vi "main.vi"() -> ()   [LabVIEW 2015]
uses:
  Solution/Controls/Zone Setup.ctl
  Solution/Controls/Zone.ctl
  Solution/Controls/Zone Indicators.ctl
  controls/state.ctl
  controls/sprinkler data.ctl
  controls/timer state.ctl
panel:
  out "error out":errorcluster
  in  "error in":errorcluster
  out "Controller Status":string
  in  "Simulation Controls":T1 {"Water Pressure Sensor (%)" scale=0.0..100.0}
  out "Zone Indicators":T2 {"Timing" format="%#.0g"}
  in  "Zone Setup Array":T3[](array[typedef])
  in  "Controls":T5
  # "Rain"
  # "No Rain"
  # "Continuous"
  # "Single"
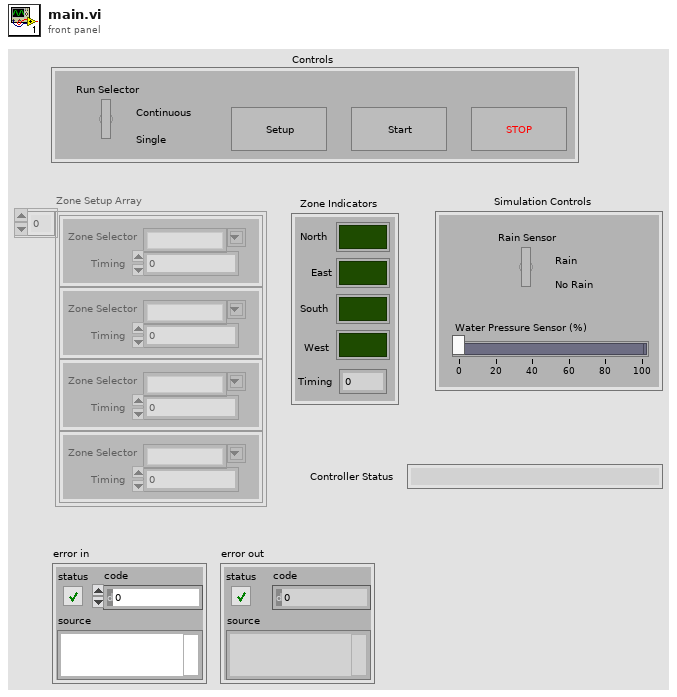
[diagram p1: front panel]
types:
  T1 = cluster{"Rain Sensor":bool, "Water Pressure Sensor (%)":dbl}
  T2 = typedef "Zone Indicators.ctl" = cluster{"North":bool, "East":bool, "South":bool, "West":bool, "Timing":dbl}
  T3 = typedef "Zone Setup.ctl" = cluster{"Zone Selector":T4, "Timing":u32}
  T4 = typedef "Zone.ctl" = string
  T5 = cluster{"Run Selector":bool, "Setup":bool, "Start":bool, "Stop":bool}
  T6 = typedef "state.ctl" = enum16{"Error", "End", "Start", "Exit", "Setup", "Low pressure", "Rain", "Run", "Idle", "Initialize"}
  T7 = enum8{"Enabled", "Disabled", "Disabled and Grayed Out"}
  T8 = typedef "timer state.ctl" = enum16{"Stop", "Start"}
  T9 = typedef "sprinkler data.ctl" = cluster{"Zone Setup Array":T3[], "Zone Indicators":T2, "order num":i32}
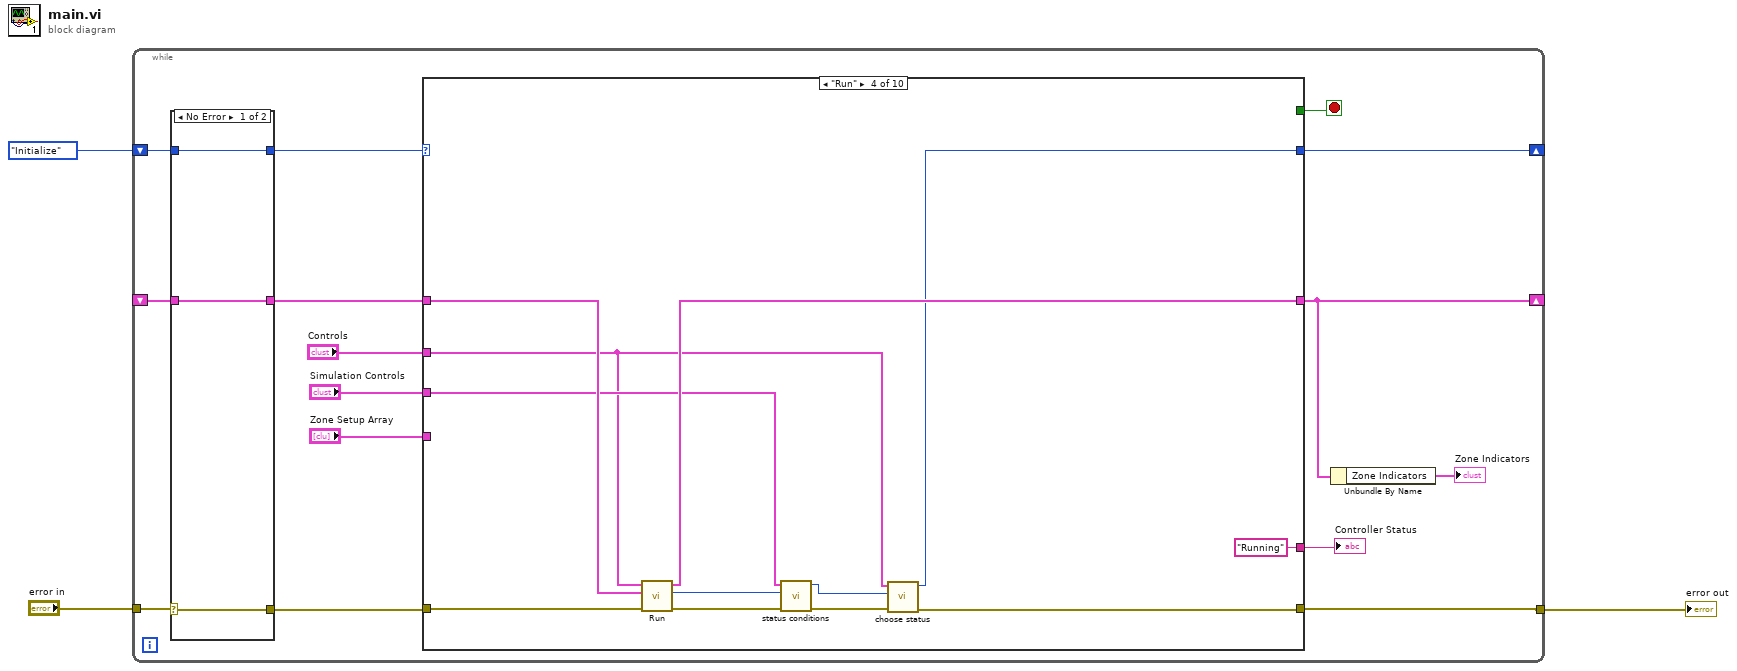
[diagram p0: block diagram]
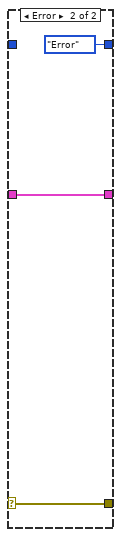
[diagram p2: hidden frame]
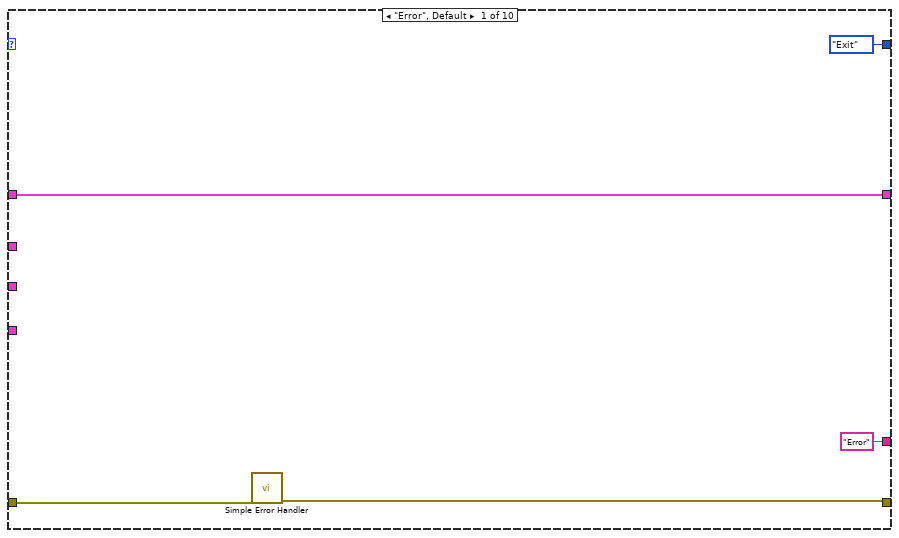
[diagram p3: hidden frame]
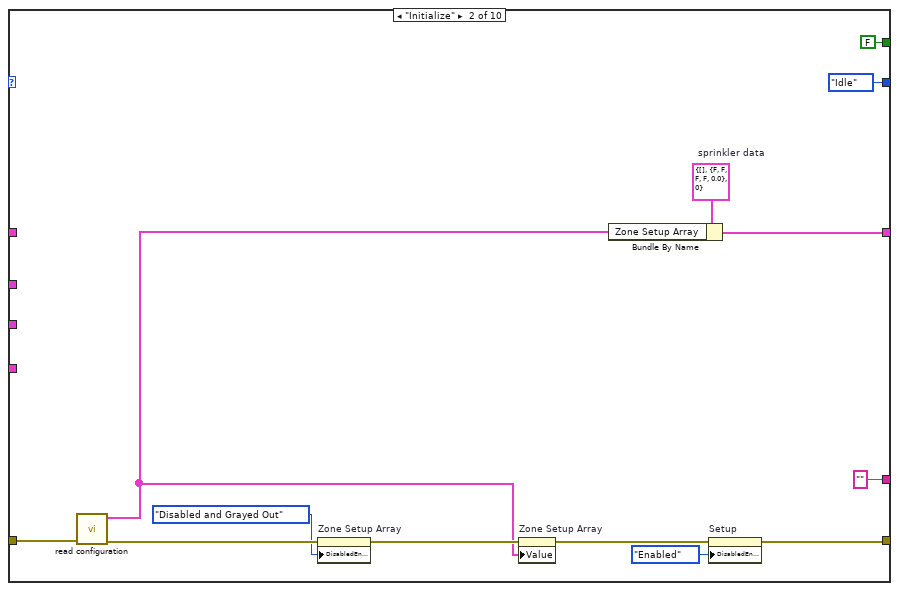
[diagram p4: hidden frame]
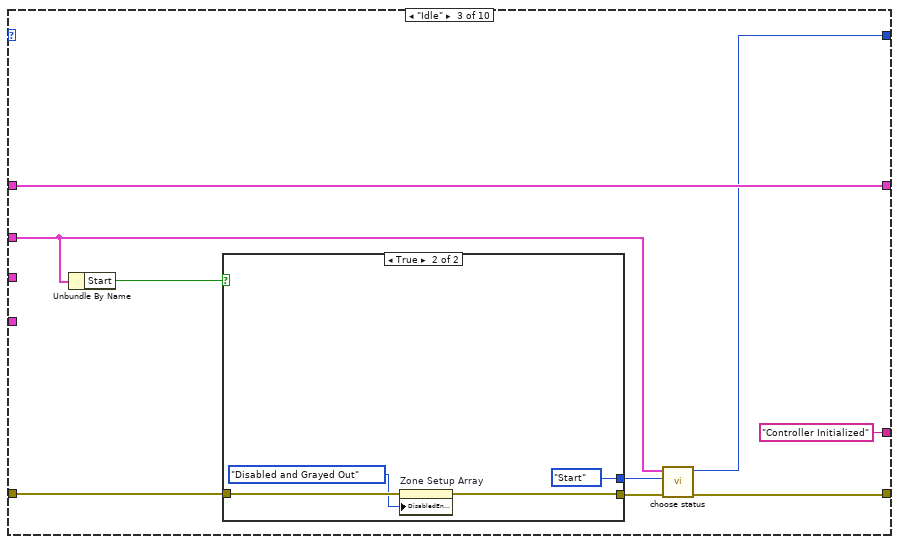
[diagram p5: hidden frame]
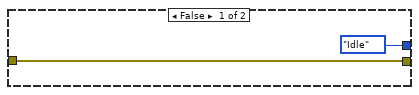
[diagram p6: hidden frame]
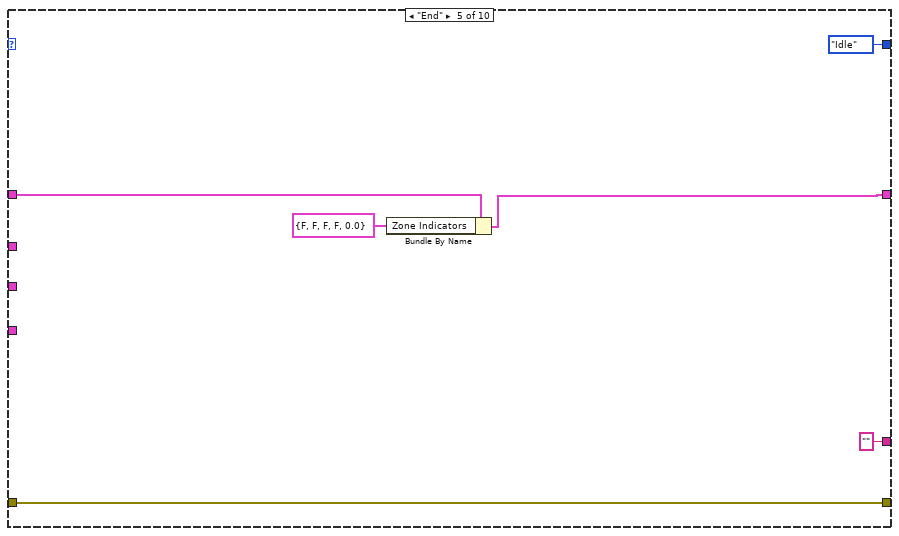
[diagram p7: hidden frame]
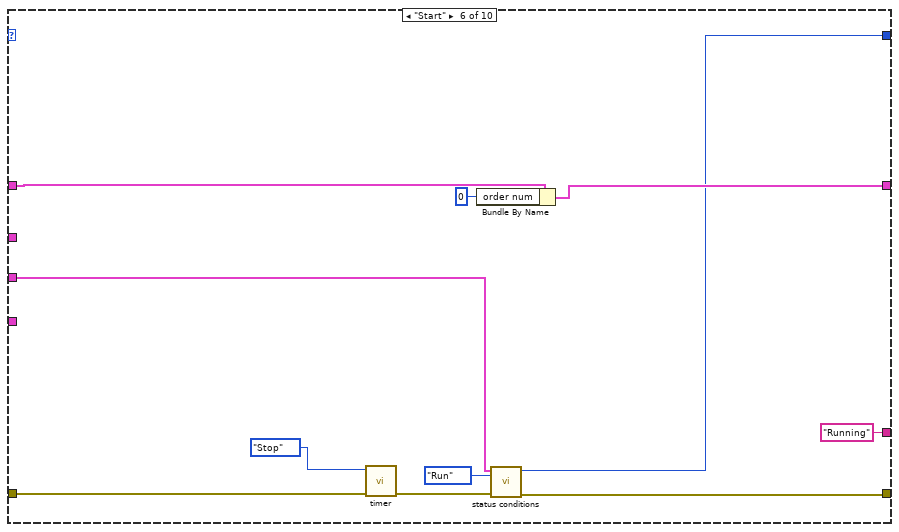
[diagram p8: hidden frame]
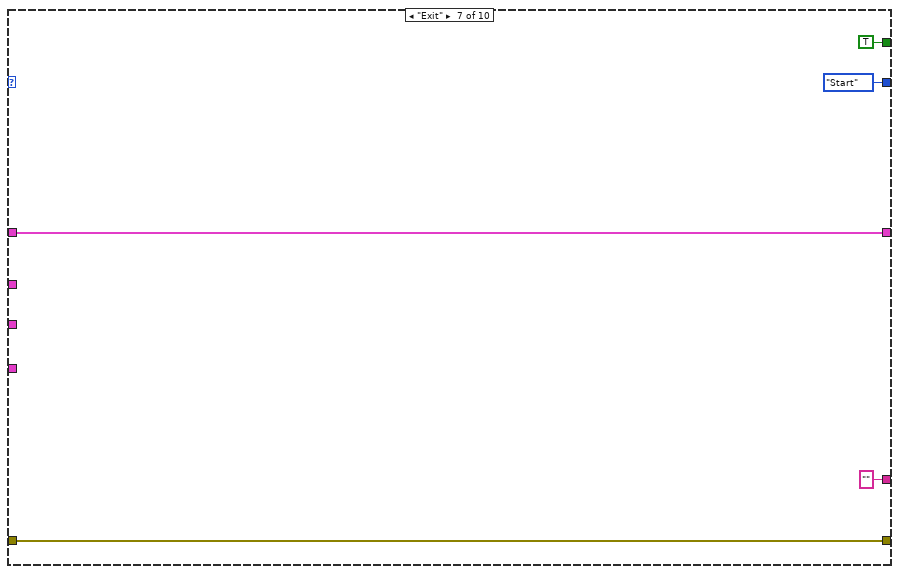
[diagram p9: hidden frame]
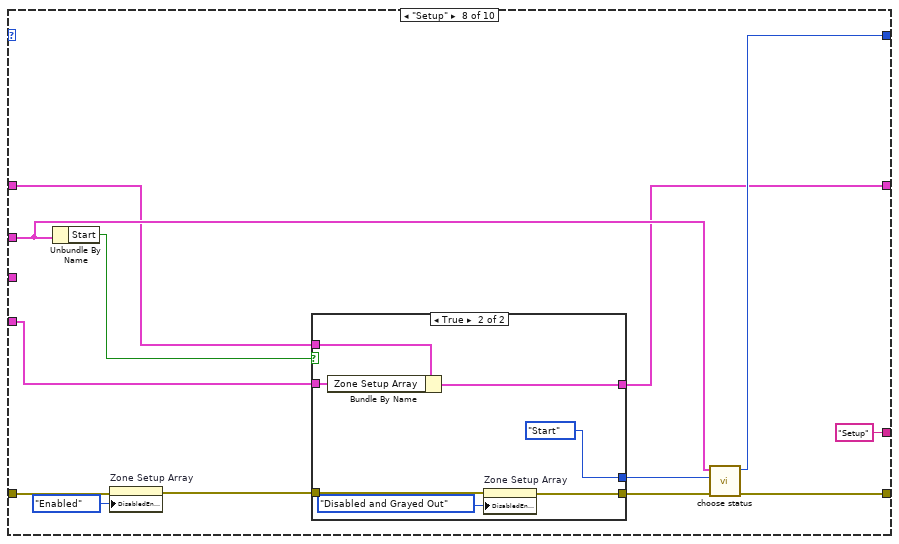
[diagram p10: hidden frame]
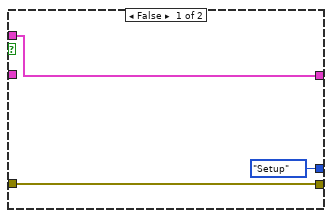
[diagram p11: hidden frame]
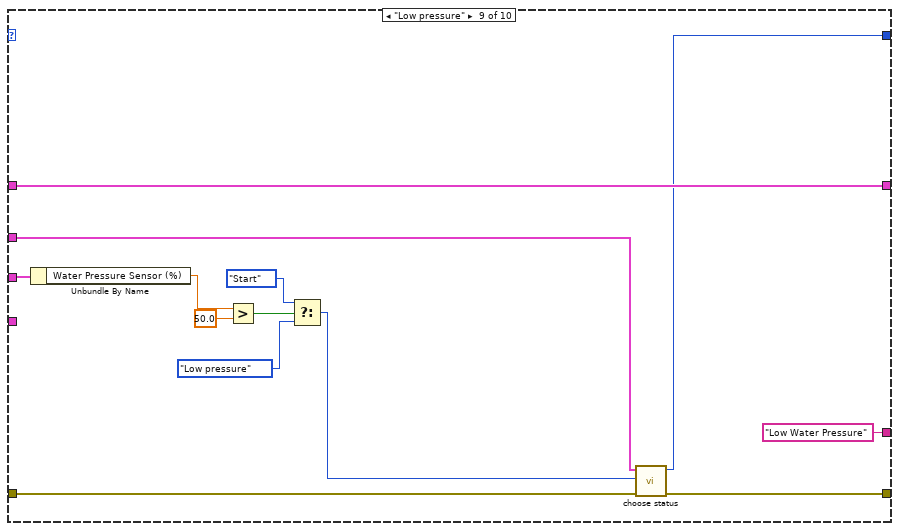
[diagram p12: hidden frame]
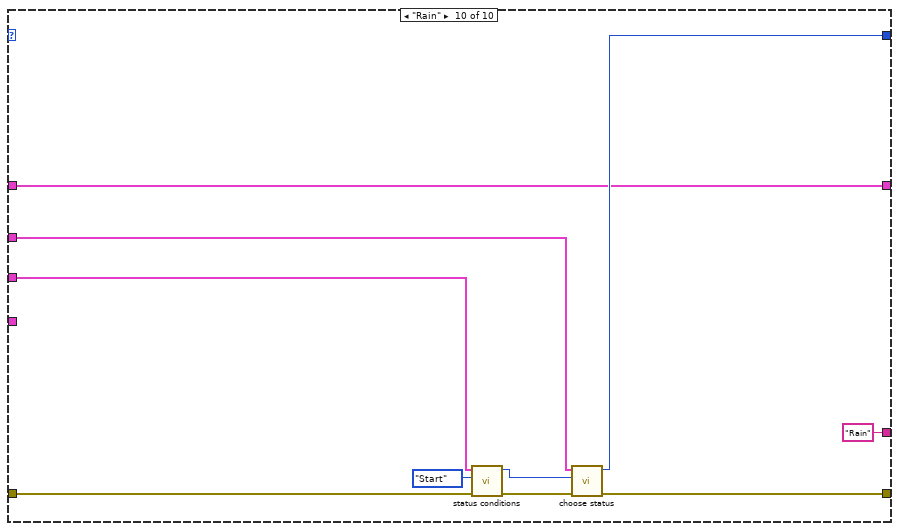
[diagram p13: hidden frame]
diagram:
  n1 = while {
    shift-right: [w13] -> _
    shift-left: state."Initialize" ("status") -> [w7]
    tunnel: "error in" -> [w10]
    tunnel: [w18] -> w1
    shift-right: [w12] -> _
    shift-left: _ -> [w8]
    stop <- w17 stop-if-true
    n2 = case shown="No Error" w10 {
      selector: w10 -> [w19 w23]
      tunnel: [w21 w24] -> w9
      tunnel: w8 -> [w21 w24]
      tunnel: w7 -> [w20 _]
      tunnel: [w20 state."Error" ("status out")] -> w6
      tunnel: [w19 w23] -> w5
      frame No Error {
      }
      frame Error {
      }
    }
    n3 = case shown="\"Run\"" w6 {
      tunnel: w5 -> [w29 w41 w50 w69 w70 w86 w88 w104 w127 w137]
      tunnel: [w28 w31 w47 w59 w70 w79 w88 w99 w126 w135] -> w18
      tunnel: [_ FALSE _ _ _ _ TRUE _ _ _] -> w17
      tunnel: [w26 w39 w49 w67 w73 w82 w89 w93 w123 w128] -> w12
      tunnel: ["Error" "" "Controller Initialized" "Running" "" "Running" "" "Setup" "Low Water Pressure" "Rain"] -> w16
      tunnel: w9 -> [w26 _ w49 w68 w75 w84 w89 w95 w123 w128]
      tunnel: "Controls" -> [_ _ w44 w62 _ _ _ w97 w124 w130]
      tunnel: "Simulation Controls" -> [_ _ _ w65 _ w78 _ _ w122 w133]
      tunnel: [state."Exit" ("status out") state."Idle" ("status out") w46 w60 state."Idle" ("status out") w76 state."Start" ("status out") w96 w115 w129] -> w13
      tunnel: "Zone Setup Array" -> [_ _ _ _ _ _ _ w94 _ _]
      frame "Error", Default {
        n4 = call <vilib>:"Simple Error Handler.vi"("error in (no error)"=w29) -> ("error out"=w28:errorcluster)  [unwired: 4 in, 4 out]
      }
      frame "Initialize" {
        w40 = T9 {"Zone Setup Array"=[], "Zone Indicators"={"North"=FALSE, "East"=FALSE, "South"=FALSE, "West"=FALSE, "Timing"=0.0}, "order num"=0}  # sprinkler data
        n5 = call "read configuration.vi"("error in (no error)"=w41) -> ("error out"=w38:errorcluster, "Zone Setup Array"=w33:T3[])  [unwired: 9 in]
        n6 = property on="Zone Setup Array" class="Arr (strict)"(error in=w38, "DisabledEnum"=T7."Disabled and Grayed Out" ("Disabled")) -> (error out=w34:errorcluster)  [unwired: 1 in, 1 out]
        n7 = property on="Zone Setup Array" class="Arr (strict)"(error in=w34, "Value"=w33) -> (error out=w32:errorcluster)  [unwired: 1 in, 1 out]
        n8 = Bundle By Name(cluster=w40, "Zone Setup Array"=w33) -> (w39:T9)
        n9 = property on="Setup" class="Bool"(error in=w32, "DisabledEnum"=T7."Enabled" ("Disabled")) -> (error out=w31:errorcluster)  [unwired: 1 in, 1 out]
      }
      frame "Idle" {
        n10 = Unbundle By Name(w44) -> ("Start"=w43:bool)
        n11 = case shown="True" w43 {
          tunnel: w50 -> [w52 w56]
          tunnel: [state."Idle" ("status") state."Start" ("status")] -> w45
          tunnel: [w52 w54] -> w48
          frame False {
          }
          frame True {
            n12 = property on="Zone Setup Array" class="Arr (strict)"(error in=w56, "DisabledEnum"=T7."Disabled and Grayed Out" ("Disabled")) -> (error out=w54:errorcluster)  [unwired: 1 in, 1 out]
          }
        }
        n13 = call "choose status.vi"("error in"=w48, "status in"=w45, "Controls"=w44) -> ("error out"=w47:errorcluster, "status out"=w46:T6)  [unwired: 7 in]
      }
      frame "Run" {
        n14 = call "Run.vi"("error in (no error)"=w69, "sprinkler data"=w68, "Controls"=w62) -> ("error out"=w66:errorcluster, "status"=w64:T6, "sprinkler data out"=w67:T9)  [unwired: 6 in]
        n15 = call "status conditions.vi"("error in"=w66, "status"=w64, "Simulation Controls"=w65) -> ("error out"=w61:errorcluster, "status out"=w63:T6)  [unwired: 7 in]
        n16 = call "choose status.vi"("error in"=w61, "status in"=w63, "Controls"=w62) -> ("error out"=w59:errorcluster, "status out"=w60:T6)  [unwired: 7 in]
      }
      frame "End" {
        n17 = Bundle By Name(cluster=w75, "Zone Indicators"=T2 {"North"=FALSE, "East"=FALSE, "South"=FALSE, "West"=FALSE, "Timing"=0.0}) -> (w73:T9)
      }
      frame "Start" {
        n18 = call "timer.vi"("error in"=w86, "timer state"=timer_state."Stop") -> ("error out"=w80:errorcluster)  [unwired: 7 in, 2 out]
        n19 = Bundle By Name(cluster=w84, "order num"=0) -> (w82:T9)
        n20 = call "status conditions.vi"("error in"=w80, "status"=state."Run" ("status out"), "Simulation Controls"=w78) -> ("error out"=w79:errorcluster, "status out"=w76:T6)  [unwired: 7 in]
      }
      frame "Exit" {
      }
      frame "Setup" {
        n21 = Unbundle By Name(w97) -> ("Start"=w101:bool)
        n22 = property on="Zone Setup Array" class="Arr (strict)"(error in=w104, "DisabledEnum"=T7."Enabled" ("Disabled")) -> (error out=w102:errorcluster)  [unwired: 1 in, 1 out]
        n23 = case shown="True" w101 {
          tunnel: w102 -> [w105 w113]
          tunnel: [w105 w112] -> w100
          tunnel: [state."Setup" ("status out") state."Start" ("status out")] -> w98
          tunnel: w95 -> [w107 w110]
          tunnel: w94 -> [_ w109]
          tunnel: [w107 w108] -> w93
          frame False {
          }
          frame True {
            n24 = Bundle By Name(cluster=w110, "Zone Setup Array"=w109) -> (w108:T9)
            n25 = property on="Zone Setup Array" class="Arr (strict)"(error in=w113, "DisabledEnum"=T7."Disabled and Grayed Out" ("Disabled")) -> (error out=w112:errorcluster)  [unwired: 1 in, 1 out]
          }
        }
        n26 = call "choose status.vi"("error in"=w100, "status in"=w98, "Controls"=w97) -> ("error out"=w99:errorcluster, "status out"=w96:T6)  [unwired: 7 in]
      }
      frame "Low pressure" {
        n27 = Unbundle By Name(w122) -> ("Water Pressure Sensor (%)"=w121:dbl)
        n28 = Greater?(x=w121, y=50.0) -> (0:w119:bool)
        n29 = Select(t=state."Start" ("status"), s=w119, f=state."Low pressure" ("status")) -> (s? t:f=w116:T6)
        n30 = call "choose status.vi"("error in"=w127, "status in"=w116, "Controls"=w124) -> ("error out"=w126:errorcluster, "status out"=w115:T6)  [unwired: 7 in]
      }
      frame "Rain" {
        n31 = call "status conditions.vi"("error in"=w137, "status"=state."Start", "Simulation Controls"=w133) -> ("error out"=w136:errorcluster, "status out"=w131:T6)  [unwired: 7 in]
        n32 = call "choose status.vi"("error in"=w136, "status in"=w131, "Controls"=w130) -> ("error out"=w135:errorcluster, "status out"=w129:T6)  [unwired: 7 in]
      }
    }
    "Controller Status" <- w16
    n33 = Unbundle By Name(w12) -> ("Zone Indicators"=→"Zone Indicators":T2)
  }
  "error out" <- w1
